vi "CheckIclRunning.vi"(8 "error in (no error)":errorcluster) -> (0 "error out":errorcluster, 3 "icl.exe running":bool)   [LabVIEW 2023, in "horiba.lvlib" / "DeviceManager.lvlib"]
uses:
  DeviceManager.lvlib
panel:
  out "offset past match":i32
  out "standard output":string
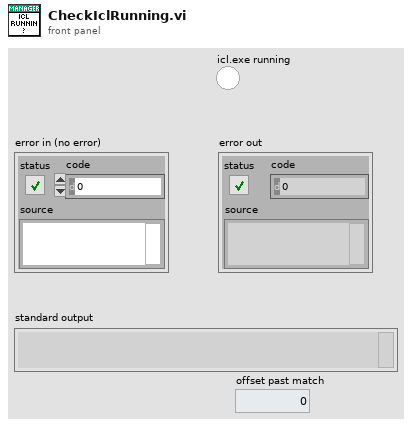
[diagram p1: front panel]
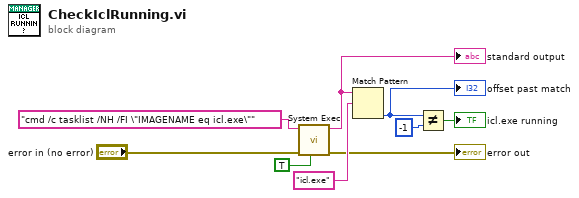
[diagram p0: block diagram]
diagram:
  n1 = call <vilib>:"System Exec.vi"("run minimized? (F)"=TRUE, "error in (no error)"="error in (no error)", "command line"="cmd /c tasklist /NH /FI \"IMAGENAME eq icl.exe\"") -> ("error out"=→"error out":errorcluster, "standard output"=w8:string)  [unwired: 5 in, 2 out]
  "standard output" <- w8
  n2 = Match Pattern(string=w8, regular expression="icl.exe") -> (offset past match=w6:i32)  [unwired: 1 in, 3 out]
  "offset past match" <- w6
  n3 = Not Equal?(x=w6, y=-1) -> (x != y?=→"icl.exe running":bool)
